vi "test_fsk.vi"() -> ()   [LabVIEW 2012]
uses:
  <vilib>/Analysis/2dsp.llb/1D Cross Correlation (CDB).vi
  <vilib>/Analysis/NI_AALPro.lvlib
panel:
  out "Recoverd Phase":dbl[](graph)
  out "Recovered Magnitude":dbl[](graph)
  out "Transmitted Phase":dbl[](graph)
  out "Transmitted Magnitude":dbl[](graph)
  out "Recovered SIgnal":dbl[](graph)
  out "Transmitted SIgnal":dbl[](graph)
  out "Correlation":dbl[](graph)
  out "Iterations":i32
  in  "stop":bool
  out "key bit stream":i8[](array[numeric]) caption="output bit stream"
  out "recovered bit sequence":i8[](array[numeric])
  in  "symbol phase continuity":enum16{"continuous", "discontinuous"}(ring)
  in  "filter length (symbols)":i32=8
  in  "filter parameter":dbl=0.8 format="%.2f"
  in  "pulse shaping filter (none)":T1(ring)=enum."Gaussian"
  in  "FSK deviation (Hz)":dbl=150000.0 format="%.2p"
  in  "samples per symbol (16)":i32=16
  in  "symbol rate (Hz)":dbl=500000000.0 format="%.2f"
  in  "total bits (128)":i32=128
  in  "passband bandwidth (Hz)":dbl=500000.0 format="%.2p"
  in  "carrier frequency (Hz)":dbl=434000000.0 min=-0.5 max=0.5 format="%.2f"
  out "BER":dbl
  in  "sync location uncertainty (symbols)":i32=1
  in  "Preamble Length":u32=20
  out "error out":errorcluster
  in  "Sync Words":i32[](array[numeric])=[1, 1, 1, 0, 0, 1, 0]
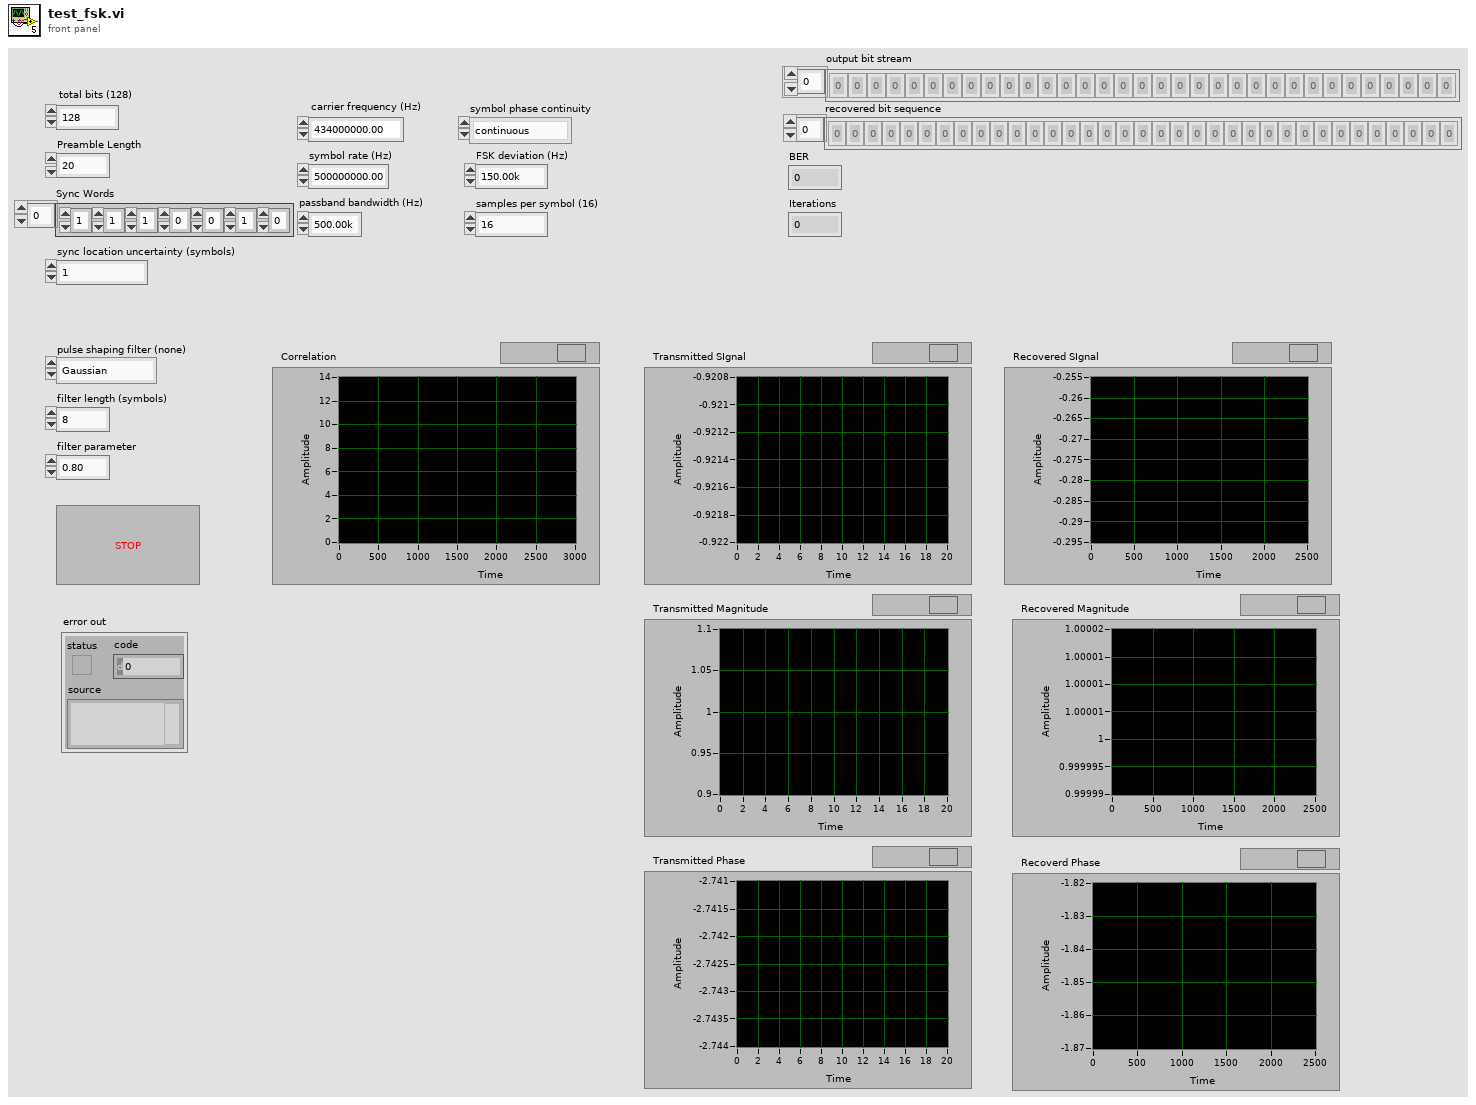
[diagram p1: front panel]
types:
  T1 = enum16{"none", "Raised Cosine", "Root Raised Cos", "Gaussian"}
  T2 = typedef "niAMT.lvlib/Complex Data Waveform.ctl" = cluster{"t0":dbl, "dt":dbl, "Y":cdb[]}
  T3 = cluster{"samples per symbol (16)":i32, "symbol map":dbl[], "symbol phase continuity":enum16{"continuous", "discontinuous"}}
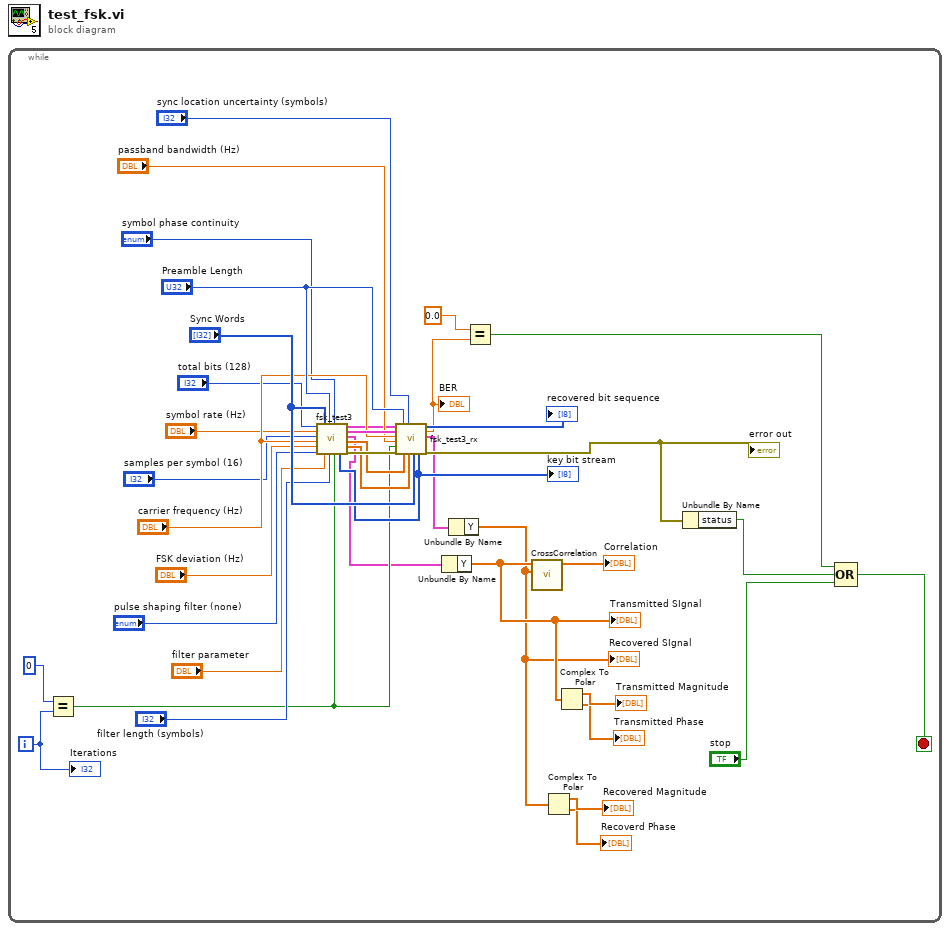
[diagram p0: block diagram]
diagram:
  n1 = while {
    i -> [w20]
    stop <- w14 stop-if-true
    n2 = Equal?(x=0, y=w20) -> (x = y?=w18:bool)
    n3 = call "fsk_test3.vi"("total bits (128)"="total bits (128)", "symbol rate (Hz)"="symbol rate (Hz)", "samples per symbol (16)"="samples per symbol (16)", "carrier frequency (Hz)"="carrier frequency (Hz)", "FSK deviation (Hz)"="FSK deviation (Hz)", "pulse shaping filter (none)"="pulse shaping filter (none)", "Sync Words"="Sync Words", "filter parameter"="filter parameter", "Preamble Length"="Preamble Length", "filter length (symbols)"="filter length (symbols)", "symbol phase continuity"="symbol phase continuity", "reset? (T)"=w18) -> ("output bit stream"=w34:i8[], "upconverted waveform (complex)"=w10:T2, "FSK system parameters"=w39:T3, "output cluster"=w7:T2, "pulse shaping filter coefficients"=w37:dbl[], "matched filter coefficients"=w36:dbl[], "error out"=w38:errorcluster)  [unwired: 1 in]
    "key bit stream" <- w34
    n4 = call "fsk_test3_rx.vi"("passband waveform (complex)"=w10, "FSK system parameters"=w39, "VCO carrier frequency (Hz)"="carrier frequency (Hz)", "passband bandwidth (Hz)"="passband bandwidth (Hz)", "reset? (F)"=w18, "error in (no error)"=w38, "expected sync location (symbols)"="Preamble Length", "pulse shaping filter coefficients"=w37, "sync location uncertainty (symbols)"="sync location uncertainty (symbols)", "matched filter coefficients"=w36, "sync bits"="Sync Words", "Key Bit Sequence"=w34) -> ("recovered bit sequence"=→"recovered bit sequence":i8[], "BER"=w13:dbl, "recovered complex waveform"=w9:T2, "error out"=w17:errorcluster)  [unwired: 4 in]
    "error out" <- w17
    "BER" <- w13
    n5 = Unbundle By Name(w7) -> ("Y"=w6:cdb[])
    "Transmitted SIgnal" <- w6
    n6 = Unbundle By Name(w9) -> ("Y"=w1:cdb[])
    "Recovered SIgnal" <- w1
    n7 = Equal?(x=0.0, y=w13) -> (x = y?=w11:bool)
    n8 = call-poly <vilib>:"CrossCorrelation.vi"("Y"=w1, "X"=w6) -> ("Rxy"=→"Correlation":cdb[])  [unwired: 8 in, 1 out]
    n9 = Complex To Polar(r * e^(i*theta)=w1) -> (r=→"Recovered Magnitude":dbl[], theta=→"Recoverd Phase":dbl[])
    n10 = Complex To Polar(r * e^(i*theta)=w6) -> (r=→"Transmitted Magnitude":dbl[], theta=→"Transmitted Phase":dbl[])
    n11 = Unbundle By Name(w17) -> ("status"=w16:bool)
    n12 = Compound Arithmetic op=OR(w11, w16, "stop") -> (w14:bool)
    "Iterations" <- w20
  }
